vi "Write Header.vi"(8 "error in (no error)":errorcluster, 10 "Header":string[](array[string]), 11 "Data Analyser Report in":refnum<class "Data Analyser Report.lvclass">) -> (0 "error out":errorcluster, 3 "Data Analyser Report out":refnum<class "Data Analyser Report.lvclass">)   [LabVIEW 2016, in "Data Analyser Report.lvclass"]
uses:
  Data Analyser Report.lvclass
  C:/Users/w.figtree/Desktop/Work/4. Projects/3. In Progress Engineering Projects/EMA/src/core/Classes/Excel Interface/Excel Sheet/Excel Sheet.lvclass
  Excel Interface/Excel Sheet/Write to Cell - String.vi
  Excel Interface/Excel Sheet/Excel Sheet.lvclass
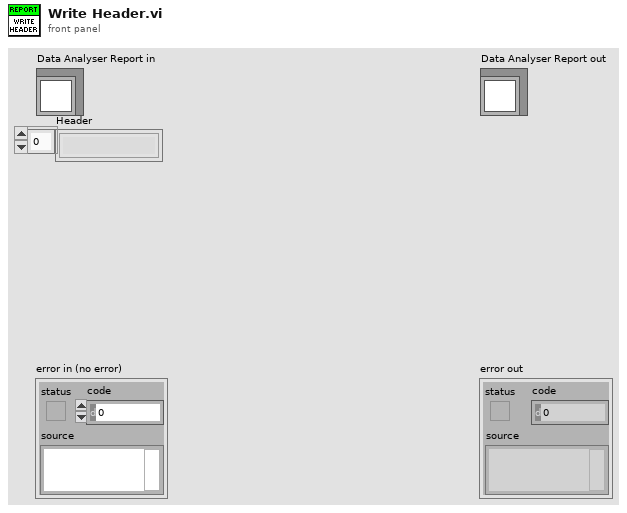
[diagram p1: front panel]
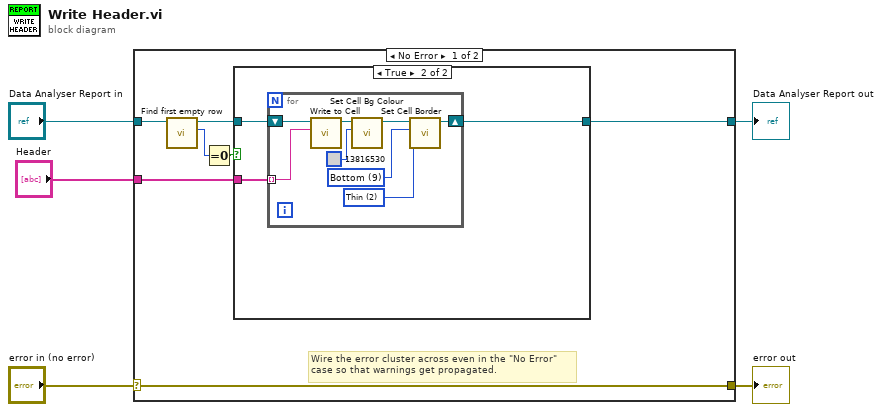
[diagram p0: block diagram]
diagram:
  n1 = case shown="No Error" "error in (no error)" {
    selector: "error in (no error)" -> [w12 w26]
    tunnel: [w12 w26] -> w4
    tunnel: [w6 w25] -> w2
    tunnel: "Data Analyser Report in" -> [w11 w25]
    tunnel: "Header" -> [w7 _]
    frame No Error {
      # "Wire the error cluster across even in the \"No Error\"\ncase so that warnings get propagated."
      n2 = call-dynamic "Find first empty row.vi"("Excel Sheet in"=w11) -> ("Next Empty Row"=w10:i32, "Excel Sheet out"=w8:refnum<class "Data Analyser Report.lvclass">)  [unwired: 8 in, 1 out]
      n3 = Equal To 0?(x=w10) -> (x = 0?=w9:bool)
      n4 = case shown="True" w9 {
        tunnel: w8 -> [w13 w16]
        tunnel: w7 -> [_ w15]
        tunnel: [w13 w14] -> w6
        frame False {
        }
        frame True {
          n5 = for {
            shift-right: [w19] -> w14
            shift-left: w16 -> [w24]
            tunnel: w15 -> [w23] mode=indexing
            w17 = 2 items=["None"=0, "Thin"=2] ("Width")
            w18 = 9 items=["Top"=8, "Bottom"=9, "Left"=7, "Right"=10] ("Edge")
            n6 = call-poly "Write to Cell.vi"("Value"=w23, "Excel Sheet in"=w24) -> ("Excel Sheet out"=w22:refnum<class "Data Analyser Report.lvclass">)  [unwired: 9 in]
            n7 = call-dynamic "Set Cell Bg Colour.vi"("Color Box"=u32 13816530, "Excel Sheet in"=w22) -> ("Excel Sheet out"=w20:refnum<class "Data Analyser Report.lvclass">)  [unwired: 9 in]
            n8 = call-dynamic "Set Cell Border.vi"("Width"=w17, "Edge"=w18, "Excel Sheet in"=w20) -> ("Excel Sheet out"=w19:refnum<class "Data Analyser Report.lvclass">)  [unwired: 8 in]
          }
        }
      }
    }
    frame Error {
    }
  }
  "error out" <- w4
  "Data Analyser Report out" <- w2
